vi "Segmentation Coin.vi"(8 "error in (no error)":errorcluster, 10 "Circle":T1, 11 "image data in":T2) -> (0 "error out":errorcluster, 3 "image data out":T2)   [LabVIEW 2017, in "image.lvlib"]
doc: "Created IvanLis by LabVIEW Portal\nProfile: http://labviewportal.org/memberlist.php?mode=viewprofile&u=987\neMail: IvanLisanov@gMail.com\nTelegram: https://t.me/IvanLis"
uses:
  image.lvlib
  <vilib>/picture/picture.llb/imagedata.ctl
  process_YOLOv8/Circle.ctl
  process_YOLOv8/process_YOLOv8.lvlib
panel:
  out "image":picture
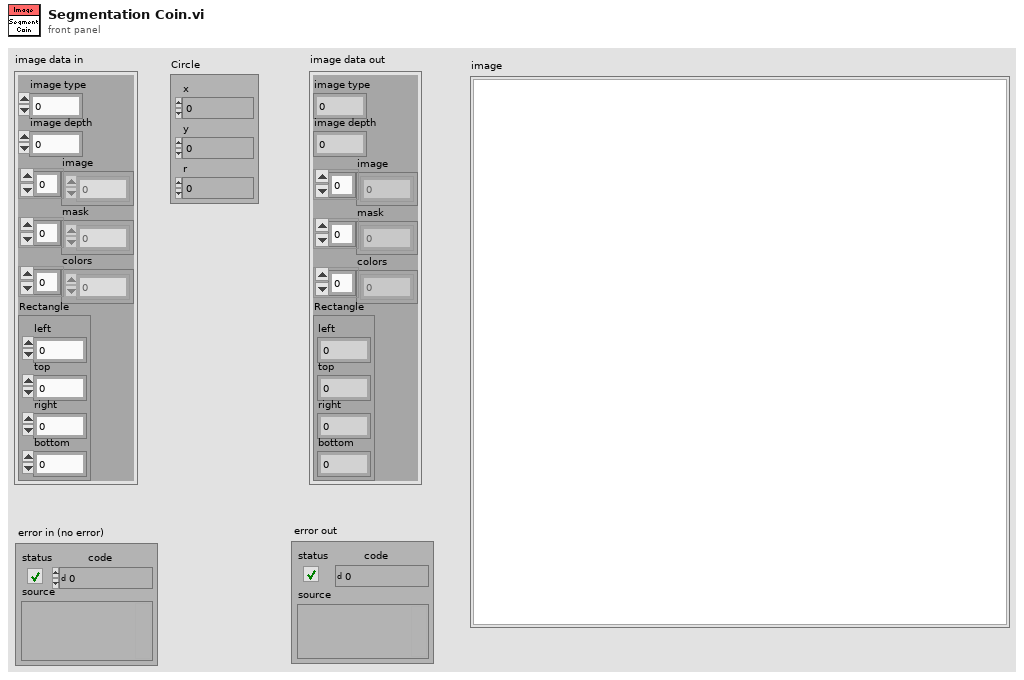
[diagram p1: front panel]
types:
  T1 = typedef "process_YOLOv8.lvlib/Circle.ctl" = cluster{"x":sgl, "y":sgl, "r":sgl}
  T2 = typedef "imagedata.ctl" = cluster{"image type":i32, "image depth":i32, "image":u8[], "mask":u8[], "colors":u32[], "Rectangle":cluster{"left":i16, "top":i16, "right":i16, "bottom":i16}}
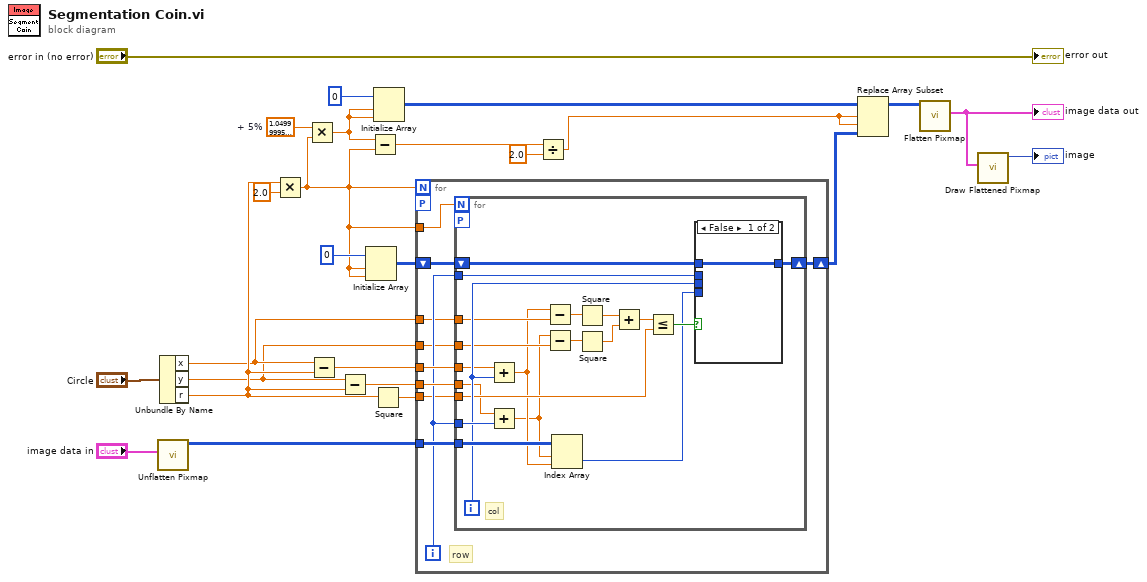
[diagram p0: block diagram]
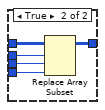
[diagram p2: hidden frame]
diagram:
  w11 = sgl 1.05  # + 5%
  n1 = call <vilib>:"Unflatten Pixmap.vi"("image data"="image data in") -> ("24-bit pixmap"=w19:u32[][])  [unwired: 10 out]
  n2 = Unbundle By Name("Circle") -> ("x"=w14:sgl, "y"=w13:sgl, "r"=w16:sgl)
  n3 = Multiply(x=w16, y=sgl 2.0) -> (x*y=w8:sgl)
  n4 = Multiply(x=w11, y=w8) -> (x*y=w9:sgl)
  n5 = Subtract(x=w14, y=w16) -> (x-y=w17:sgl)
  n6 = Subtract(x=w13, y=w16) -> (x-y=w15:sgl)
  n7 = Initialize Array(u32 0 ("element"), w8, w8) -> (w20:u32[][])
  n8 = Subtract(x=w9, y=w8) -> (x-y=w7:sgl)
  n9 = Square(x=w16) -> (x^2=w18:sgl)
  n10 = Initialize Array(u32 0 ("element"), w9, w9) -> (w6:u32[][])
  n11 = for {
    N: w8 -> [_]
    tunnel: w17 -> [w34]
    tunnel: w15 -> [w33]
    tunnel: w8 -> [w35]
    shift-right: [w31] -> w5
    shift-left: w20 -> [w32]
    tunnel: w19 -> [w30]
    tunnel: w18 -> [w28]
    tunnel: w14 -> [w27]
    tunnel: w13 -> [w26]
    workers-P: _ -> [_]
    i -> [w29]
    # "row"
    n12 = for {
      N: w35 -> [_]
      tunnel: w34 -> [w39]
      tunnel: w33 -> [w38]
      shift-right: [w55] -> w31
      shift-left: w32 -> [w54]
      tunnel: w29 -> [w51]
      tunnel: w30 -> [w53]
      tunnel: w29 -> [w52]
      tunnel: w28 -> [w44]
      tunnel: w27 -> [w41]
      tunnel: w26 -> [w40]
      workers-P: _ -> [_]
      i -> [w50]
      # "col"
      n13 = Add(x=w39, y=w50) -> (x+y=w37:sgl)
      n14 = Add(x=w38, y=w52) -> (x+y=w36:sgl)
      n15 = Subtract(x=w37, y=w41) -> (x-y=w49:sgl)
      n16 = Subtract(x=w36, y=w40) -> (x-y=w48:sgl)
      n17 = Index Array(array=w53, index (row)=w36, index (col)=w37) -> (element=w42:u32)
      n18 = Square(x=w49) -> (x^2=w47:sgl)
      n19 = Square(x=w48) -> (x^2=w46:sgl)
      n20 = Add(x=w47, y=w46) -> (x+y=w45:sgl)
      n21 = Less Or Equal?(x=w45, y=w44) -> (x <= y?=w43:bool)
      n22 = case shown="False" w43 {
        tunnel: [w56 w61] -> w55
        tunnel: w54 -> [w56 w60]
        tunnel: w51 -> [_ w59]
        tunnel: w50 -> [_ w58]
        tunnel: w42 -> [_ w57]
        frame False {
        }
        frame True {
          n23 = Replace Array Subset(array=w60, new element=w57, index (row)=w59, index (col)=w58) -> (w61:u32[][])
        }
      }
    }
  }
  n24 = Divide(x=w7, y=sgl 2.0) -> (x/y=w4:sgl)
  n25 = Replace Array Subset(array=w6, new element=w5, index (row)=w4, index (col)=w4) -> (w3:u32[][])
  n26 = call <vilib>:"Flatten Pixmap.vi"("24-bit pixmap"=w3) -> ("image data"=w1:T2)  [unwired: 6 in, 4 out]
  "image data out" <- w1
  n27 = call <vilib>:"Draw Flattened Pixmap.vi"("image data"=w1) -> ("new picture"=→"image":picture)  [unwired: 8 in]
  "error out" <- "error in (no error)"
